vi "Write Command to Execute.vi"(8 "error in (no error)":errorcluster, 10 "Command to Execute":string, 11 "User Defined Read in":refnum<class "User Defined Read.lvclass">) -> (0 "error out":errorcluster, 3 "User Defined Read out":refnum<class "User Defined Read.lvclass">)   [LabVIEW 2023, in "HAF.lvlib" / "User Defined Read.lvclass"]
doc: "Saves a new SCPI command string that this Command is responsible for running."
uses:
  User Defined Read.lvclass
  User Defined Read.lvclass/User Defined Read.ctl
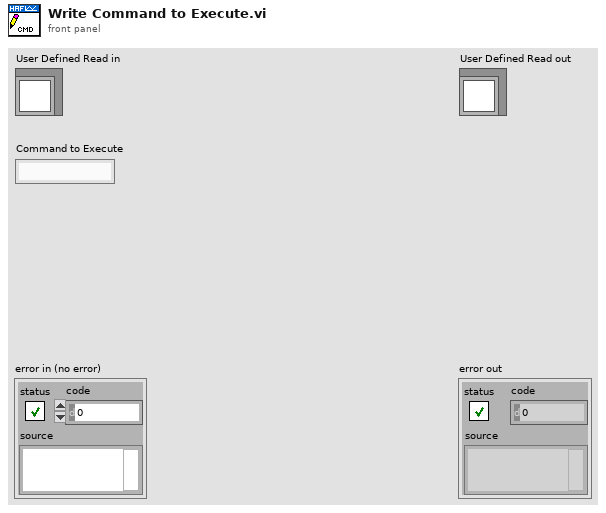
[diagram p1: front panel]
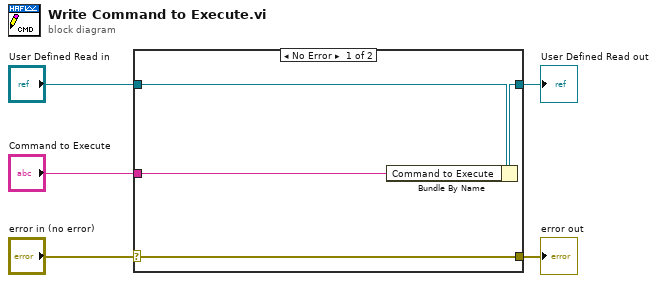
[diagram p0: block diagram]
diagram:
  n1 = case shown="No Error" "error in (no error)" {
    selector: "error in (no error)" -> [w9 w10]
    tunnel: [w9 w10] -> w4
    tunnel: [w7 w11] -> w2
    tunnel: "User Defined Read in" -> [w8 w11]
    tunnel: "Command to Execute" -> [w6 _]
    frame No Error {
      n2 = Bundle By Name(cluster=w8, "Command to Execute"=w6) -> (w7:refnum<class "User Defined Read.lvclass">)
    }
    frame Error {
    }
  }
  "error out" <- w4
  "User Defined Read out" <- w2
